vi "CloseConnection.vi"(8 "error in (no error)":errorcluster, 11 "TCP In":refnum<class "TCP.lvclass">) -> (0 "error out":errorcluster, 3 "TCP Out":refnum<class "TCP.lvclass">)   [LabVIEW 2019, in "TCP.lvclass"]
uses:
  TCP.lvclass
  TCP.lvclass/TCP.ctl
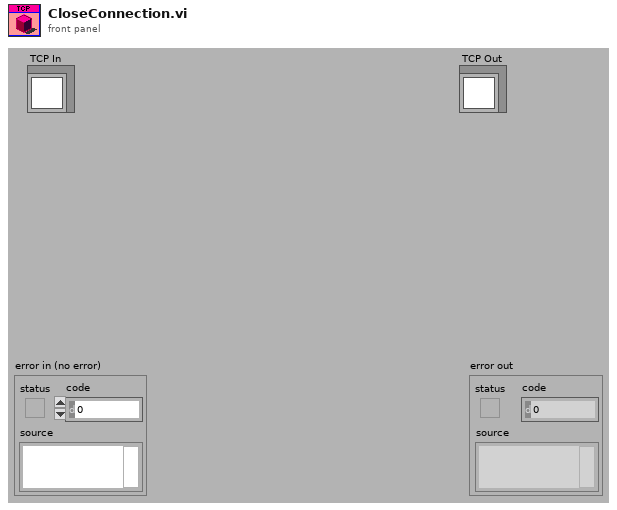
[diagram p1: front panel]
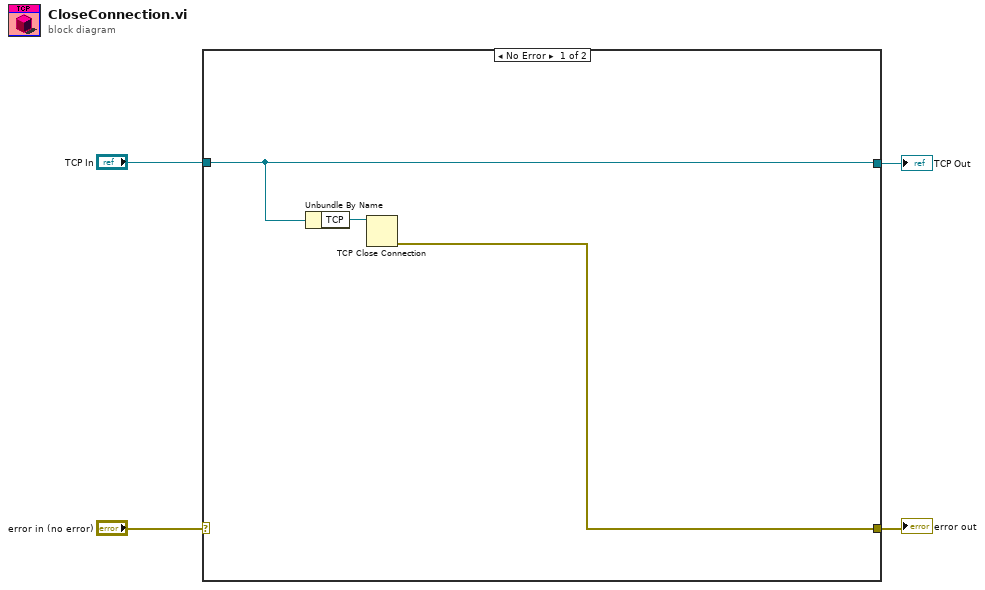
[diagram p0: block diagram]
diagram:
  n1 = case shown="No Error" "error in (no error)" {
    selector: "error in (no error)" -> [_ w9]
    tunnel: [w5 w9] -> w3
    tunnel: [w7 w8] -> w1
    tunnel: "TCP In" -> [w7 w8]
    frame No Error {
      n2 = Unbundle By Name(w7) -> ("TCP"=w6:refnum<k5>)
      n3 = TCP Close Connection(connection ID=w6) -> (error out=w5:errorcluster)  [unwired: 2 in, 1 out]
    }
    frame Error {
    }
  }
  "error out" <- w3
  "TCP Out" <- w1
